vi "art联动采集V4.8.4(导入色码表).vi"() -> ()   [LabVIEW 2016]
uses:
  <vilib>/Utility/file.llb/Read Delimited Spreadsheet (I64).vi
  <vilib>/Instr/_visa.llb/VISA Configure Serial Port (Instr).vi
  <vilib>/Utility/file.llb/Write Delimited Spreadsheet (DBL).vi
panel:
  in  "色码表导入":path caption="（色码表导入）"
  out "水平进度条":u8(slide) scale=0.0..100.0
  out "x+y 3":dbl=3.0
  in  "分层图查看":bool
  in  "hDevice 2":i32
  in  "逐行扫描":bool
  in  "定位模式":bool
  in  "X终点":dbl
  in  "Y终点":dbl
  in  "高级设置":bool
  in  "Y轴回零速度":dbl=15000.0
  in  "X轴回零速度":dbl=15000.0
  in  "细分设置":dbl=8.0
  in  "等待时间":u32=40
  in  "文件保存":path=path "C:/Users/H301/Desktop/art采集实验数据" caption="保存路径"
  out "已用时（s）":dbl
  out "error out":errorcluster caption="错误输出"
  in  "退出扫描(Esc)":bool
  in  "N_Length":i32=16384
  out "M_Length":i32
  out "hDevice":i32=241832032
  out "pulDDR2Length":u32=256
  out "毫秒计时值":u32=3586537
  out "数组":dbl[][](array[numeric])=[[58819.77200735986, 88200.32943600747]]
  out "强度图":dbl[][](graph)=[[58819.77200735986, 88200.32943600747]]
  out "judge":dbl
  out "Xloop":dbl
  out "幅频谱":dbl[](graph)
  out "时域谱":dbl[](graph)
  out "错误输出":errorcluster
  in  "启动":bool
  in  "逐点扫描":bool
  in  "X归零":bool
  in  "Y归零":bool
  in  "Y起点":dbl
  in  "Y轴速度":dbl=9000.0
  in  "X轴速度":dbl=9000.0
  out "电机状态":bool
  in  "电机端口":refnum<visa-resource-name>="COM6"
  out "Yloop":dbl=1.0
  out "X扫描范围":dbl=150.0
  out "Y扫描范围":dbl=75.0
  out "Y序":i32
  in  "X起点":dbl
  out "Y(mm)":dbl
  out "x+y 2":dbl=3.0
  in  "Y:":dbl=1.0
  in  "精度":dbl=0.001
  in  "电机急停":bool
  out "X（mm）":dbl
  out "x+y":dbl=1.0
  in  "X:":dbl=1.0
  # "实时坐标"
  # "时域谱"
  # "频域谱"
  # "归零"
  # "扫描区域"
  # "扫描步进(mm)"
  # "X:"
  # "~"
  # "Y:"
  # "~"
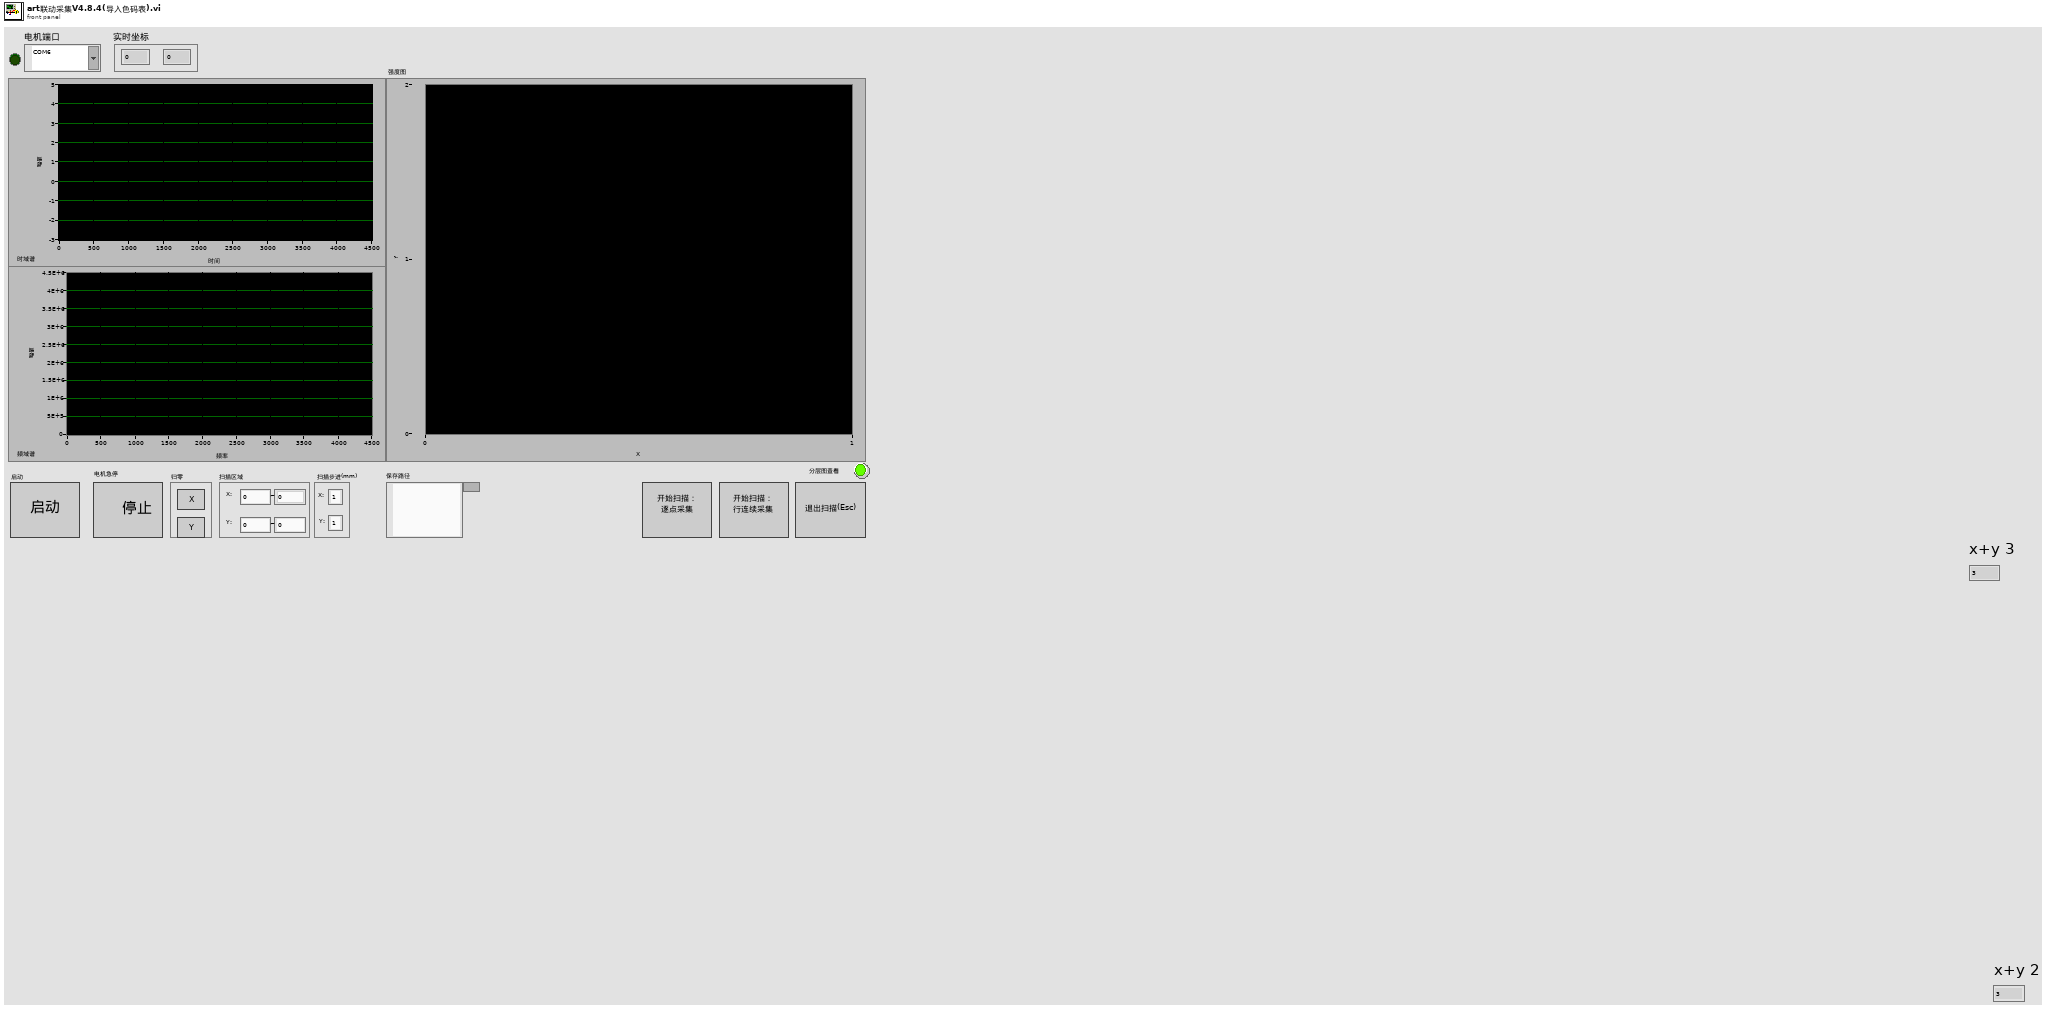
[diagram p1: front panel]
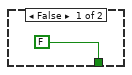
[diagram p2: hidden frame]
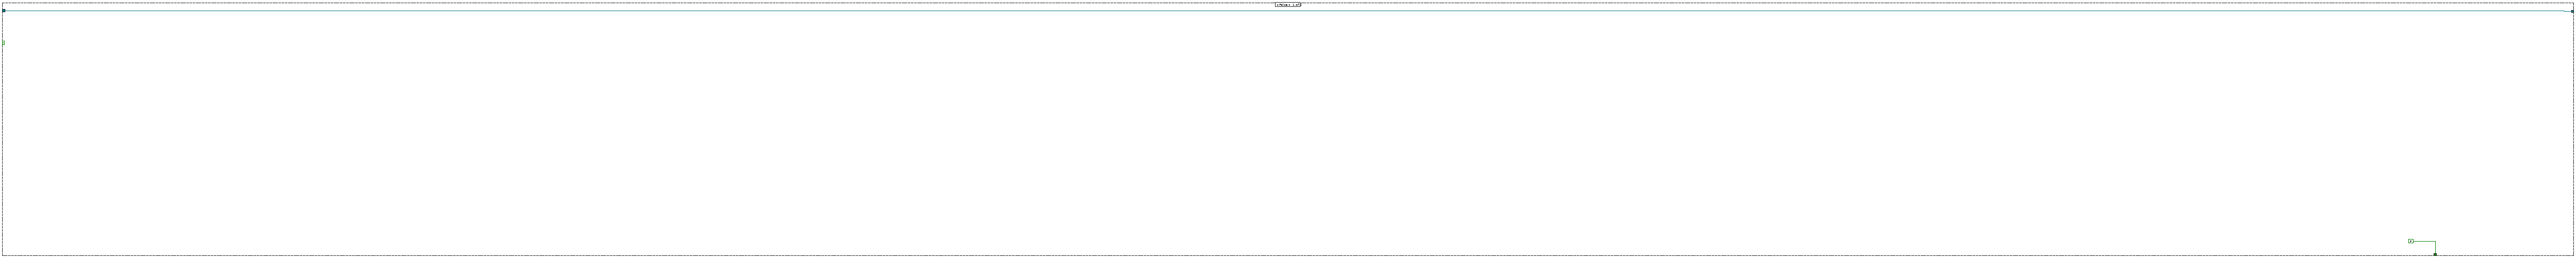
[diagram p3: hidden frame]
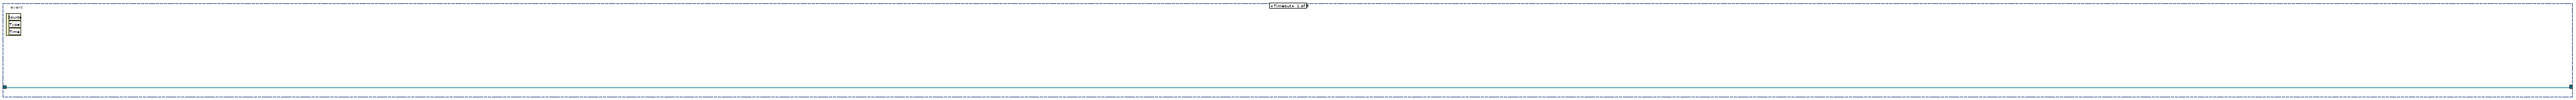
[diagram p4: hidden frame]
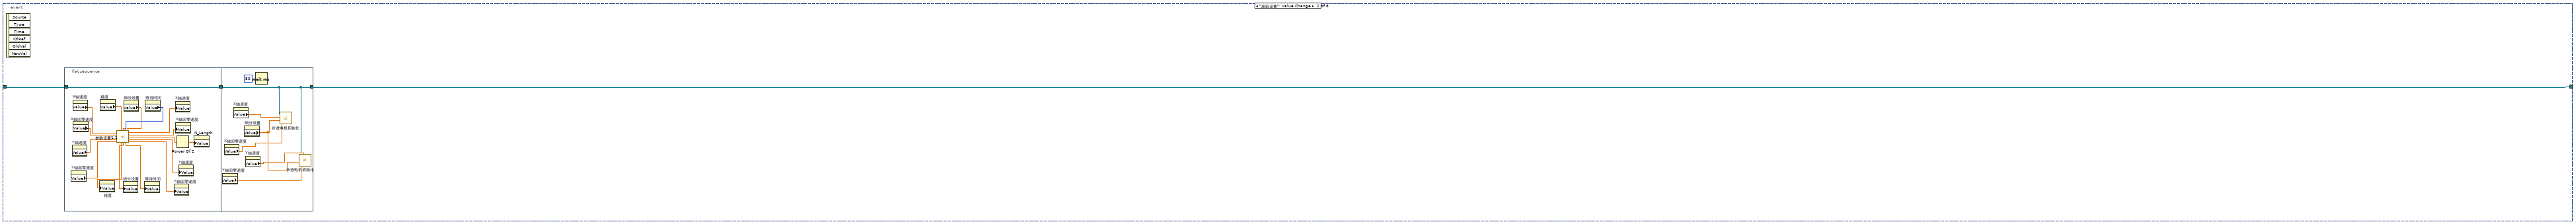
[diagram p5: hidden frame]
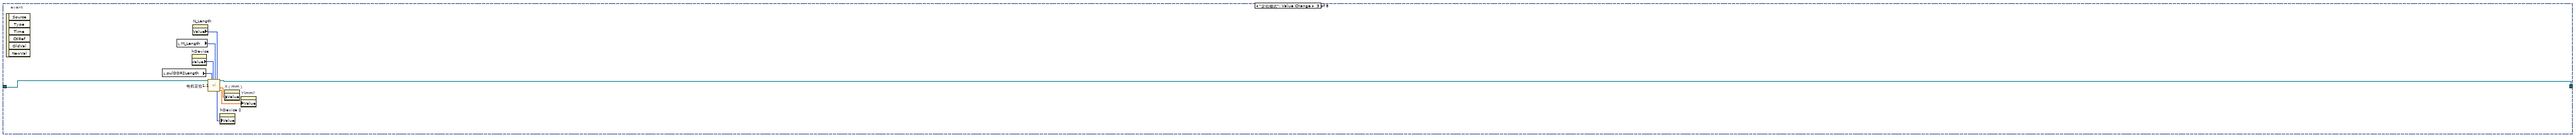
[diagram p6: hidden frame]
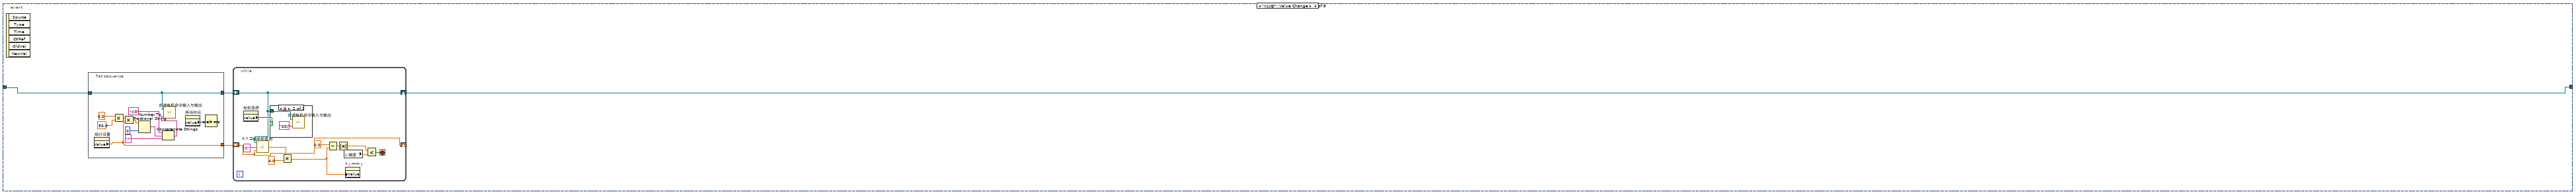
[diagram p7: hidden frame]
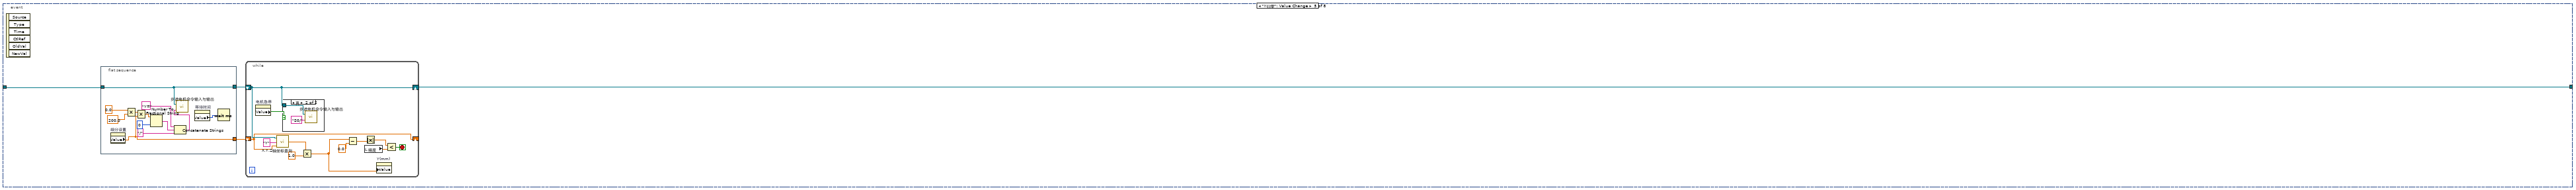
[diagram p9: hidden frame]
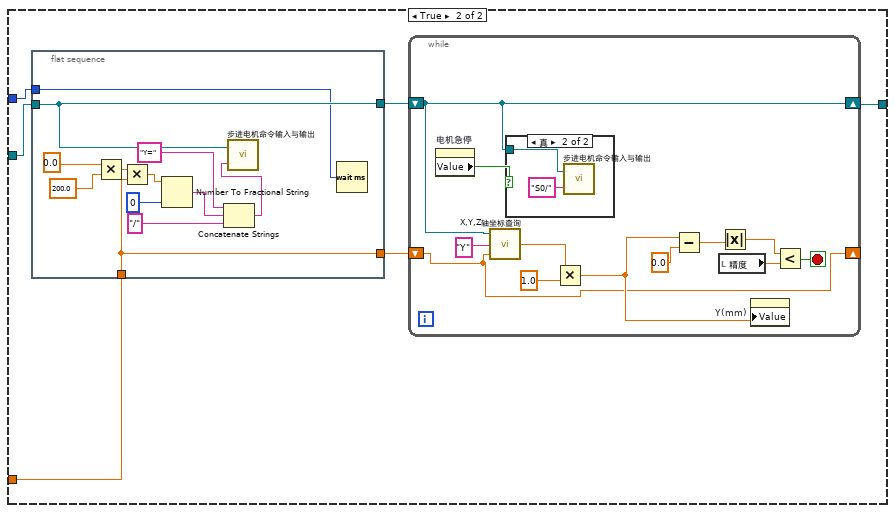
[diagram p15: hidden frame]
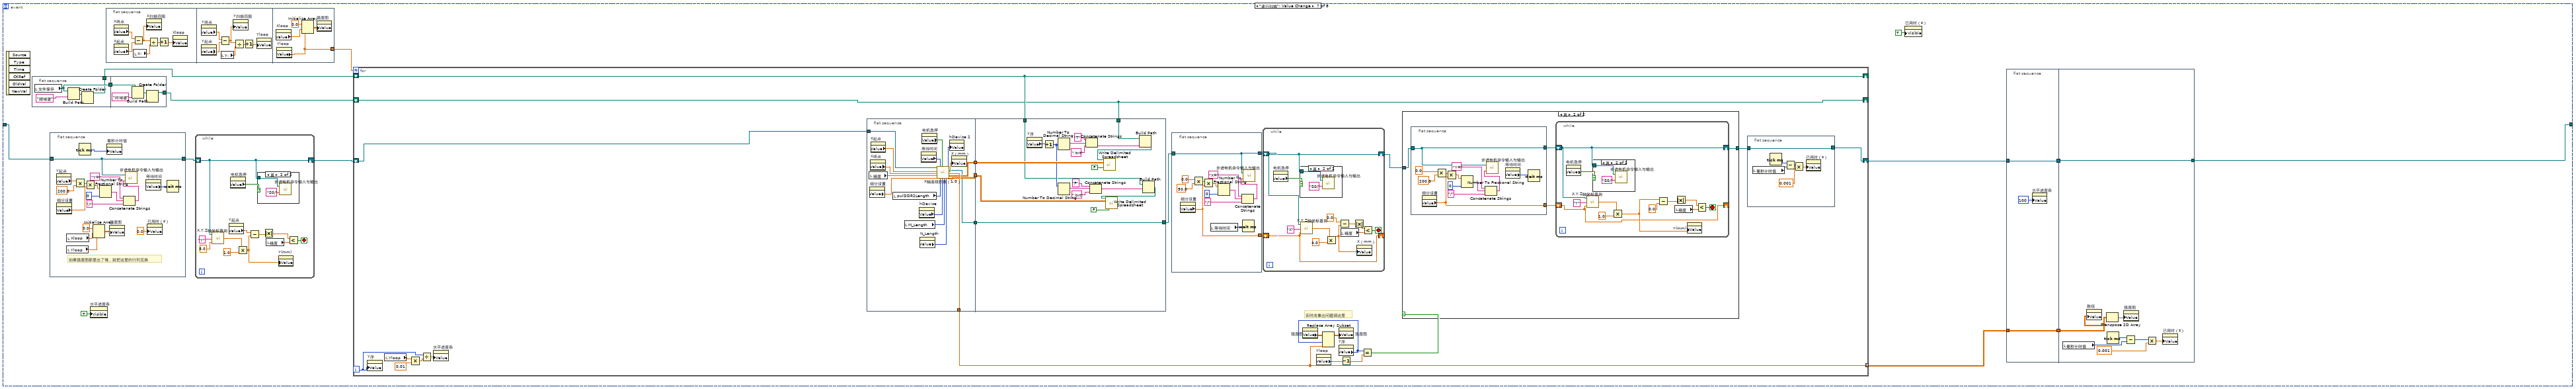
[diagram p19: hidden frame]
diagram:
  n1 = call-poly <vilib>:"Read Delimited Spreadsheet.vi"("file path (dialog if empty)"="色码表导入") -> ("first row"=w1:i64[])  [unwired: 9 in, 5 out]
  n2 = property on="强度图" class="IntGraph (严格)"("Color Table"=w1) -> ()  [unwired: 2 in, 2 out]
  n3 = property on="水平进度条" class="Slide (严格)"("Visible"=FALSE ("可见")) -> ()  [unwired: 2 in, 2 out]
  n4 = while {
    stop <- w7 stop-if-true
    n5 = case shown="真" "启动" {
      tunnel: [FALSE ("ESC") w16] -> w7
      frame False {
      }
      frame True {
        w29 = 0  # OutClockSource
        w30 = 0  # bClockSourceDir
        w32 = 10000000  # Frequency
        w33 = 0  # ClockSource
        w34 = 0  # TrigLevelVolt
        w22 = 1
        w35 = 0  # TriggerDir
        w36 = 0  # TriggerSource
        w37 = 0  # ATRTriggerChannel
        w38 = 0  # TriggerMode
        w23 = 0  # M_Length
        w39 = 1  # CouplingType
        w40 = 0  # DeviceLgcID
        w50 = u16 0 items=["无", "XON/XOFF", "RTS/CTS", "XON/XOFF & RTS/CTS", "DTR/DSR", "XON/XOFF & DTR/DSR"] ("flow control (0:none)")
        w51 = u16 10 items=["1.0"=10, "1.5"=15, "2.0"=20] ("stop bits (10: 1 bit)")
        # "3"
        # "2"
        # "1"
        n6 = call-poly "VISA Configure Serial Port"("VISA resource name"="电机端口", "baud rate (9600)"=u32 9600, "data bits (8)"=u16 8, "parity (0:none)"=enum16{"None", "Odd", "Even", "Mark", "Space"}."None", "stop bits (10: 1 bit)"=w51, "flow control (0:none)"=w50) -> ("VISA resource name out"=w42:refnum<visa-resource-name>, "error out"=→"error out":errorcluster)  [unwired: 1 in, 7 out]
        n7 = Build Array "InputRange"(w22, w22, w22, w22) -> (w21:i32[])
        n8 = dll-call lib="PTH2aabs CUsersH301Desktopart闭环扫描程序采集卡控制INFamd64PCI8502_32.dll" fn="PCI8502_CreateDevice" label="CreateDevice"("DeviceLgcID"=w40) -> (w27:i32)  [unwired: 4 in, 2 out]
        n9 = property on="细分设置" class="DigNum (严格)"() -> ("Value"=w15:dbl)  [unwired: 2 in, 2 out]
        n10 = Build Array (concatenate) "InitDeviceAD"(w32, w21, w39, w23, "N_Length", w38, w37, w36, w35, w34, w33, w30, w29) -> (w31:i32[])
        n11 = call "步进电机初始化.vi"("回零速度"="X轴回零速度", "细分设置"=w15, "X轴速度"="X轴速度", "串口通信端口"=w42) -> ()  [unwired: 2 in, 1 out]
        n12 = dll-call lib="PTH2aabs CUsersH301Desktopart闭环扫描程序采集卡控制INFamd64PCI8502_32.dll" fn="PCI8502_GetDDR2Length" label="GetDDR2Length"("hDevice"=w27, "pulDDR2Length"=u32 0) -> ("hDevice"=w26:i32, "pulDDR2Length"=→"pulDDR2Length":u32)  [unwired: 4 in, 2 out]
        n13 = call "步进电机初始化.vi"("Y轴速度"="Y轴速度", "回零速度"="Y轴回零速度", "细分设置"=w15, "串口通信端口"=w42) -> ()  [unwired: 2 in, 1 out]
        n14 = call "步进电机命令输入与输出.vi"("输入字符串"="?R/", "串口通信端口"=w42) -> ("返回字符串"=w47:string)
        n15 = dll-call lib="PTH2aabs CUsersH301Desktopart闭环扫描程序采集卡控制INFamd64PCI8502_32.dll" fn="PCI8502_InitDeviceAD" label="InitDeviceAD"("hDevice"=w26, "pADPara"=w31) -> ("hDevice"=→"hDevice":i32)  [unwired: 5 in, 2 out]
        n16 = String Subset(string=w47, offset (0)=0 ("偏移量(0)"), length (rest)=2 ("长度（剩余）")) -> (substring=w44:string)
        n17 = Equal?(x=w44, y="OK") -> (x = y?=w41:bool)
        "电机状态" <- w41
        n18 = case shown="真" w41 {
          tunnel: w42 -> [w57 w60]
          tunnel: [w57 w58] -> w17
          tunnel: [FALSE ("ESC") w59] -> w16
          frame False {
          }
          frame True {
            n19 = while {
              tunnel: ["退出扫描(Esc)"] -> w59
              shift-right: [w63] -> w58
              shift-left: w60 -> [w68]
              stop <- "退出扫描(Esc)" stop-if-true
              n20 = property on="水平进度条" class="Slide (严格)"("Visible"=FALSE ("可见")) -> ()  [unwired: 2 in, 2 out]
              n21 = property on="高级设置" class="Bool"("Visible"=TRUE ("可见")) -> ()  [unwired: 2 in, 2 out]
              n22 = property on="定位模式" class="Bool"("Visible"=TRUE ("可见")) -> ()  [unwired: 2 in, 2 out]
              n23 = property on="水平进度条" class="Slide (严格)"("Value"=u8 0 ("水平进度条")) -> ()  [unwired: 2 in, 2 out]
              n24 = event shown="[5] \"逐点扫描\": 值改变" {
                selector: _ -> [_ _ _ _ _ _ _ _]
                dyn-events: _ -> [_ _ _ _ _ _ _ _]
                timeout: 1 -> [_ _ _ _ _ _ _ _]
                tunnel: w68 -> [w69 w72 w105 w109 w139 w190 w499 w727]
                tunnel: [w69 w71 w104 w107 w137 w185 w502 w726] -> w63
                event Timeout {
                  n25 = event-data() -> ()  [unwired: 1 in, 3 out]
                }
                event "高级设置": Value Change {
                  n26 = event-data() -> ()  [unwired: 1 in, 6 out]
                  n27 = flat-sequence {
                    tunnel: w72 -> [w75]
                    tunnel: [w75] -> w70
                    tunnel: [w91] -> w71
                    tunnel: w70 -> [w91]
                    frame #0 {
                      n28 = property on="Y轴回零速度" class="DigNum (严格)"() -> ("Value"=w79:dbl)  [unwired: 2 in, 2 out]
                      n29 = property on="Y轴速度" class="DigNum (严格)"() -> ("Value"=w78:dbl)  [unwired: 2 in, 2 out]
                      n30 = property on="X轴速度" class="DigNum (严格)"() -> ("Value"=w76:dbl)  [unwired: 2 in, 2 out]
                      n31 = property on="X轴回零速度" class="DigNum (严格)"() -> ("Value"=w77:dbl)  [unwired: 2 in, 2 out]
                      n32 = property on="精度" class="DigNum (严格)"() -> ("Value"=w83:dbl)  [unwired: 2 in, 2 out]
                      n33 = property on="细分设置" class="DigNum (严格)"() -> ("Value"=w84:dbl)  [unwired: 2 in, 2 out]
                      n34 = property on="等待时间" class="DigNum (严格)"() -> ("Value"=w85:u32)  [unwired: 2 in, 2 out]
                      n35 = call "参数设置1.1.vi"("X轴速度"=w76, "精度"=w83, "细分设置"=w84, "等待时间"=w85, "X轴回零速度"=w77, "Y轴速度"=w78, "Y轴回零速度"=w79) -> ("X轴速度"=w86:dbl, "X轴回零速度"=w87:dbl, "采样阶"=w73:dbl, "Y轴速度"=w88:dbl, "精度"=w80:dbl, "细分设置"=w81:dbl, "等待时间"=w82:dbl, "Y轴回零速度"=w89:dbl)  [unwired: 1 in]
                      n36 = property on="精度" class="DigNum (严格)"("Value"=w80) -> ()  [unwired: 2 in, 2 out]
                      n37 = property on="细分设置" class="DigNum (严格)"("Value"=w81) -> ()  [unwired: 2 in, 2 out]
                      n38 = property on="等待时间" class="DigNum (严格)"("Value"=w82) -> ()  [unwired: 2 in, 2 out]
                      n39 = property on="Y轴回零速度" class="DigNum (严格)"("Value"=w89) -> ()  [unwired: 2 in, 2 out]
                      n40 = property on="X轴速度" class="DigNum (严格)"("Value"=w86) -> ()  [unwired: 2 in, 2 out]
                      n41 = property on="X轴回零速度" class="DigNum (严格)"("Value"=w87) -> ()  [unwired: 2 in, 2 out]
                      n42 = Power Of 2(x=w73) -> (2^x=w74:dbl)
                      n43 = property on="Y轴速度" class="DigNum (严格)"("Value"=w88) -> ()  [unwired: 2 in, 2 out]
                      n44 = property on="N_Length" class="DigNum (严格)"("Value"=w74) -> ()  [unwired: 2 in, 2 out]
                    }
                    frame #1 {
                      n45 = property on="Y轴回零速度" class="DigNum (严格)"() -> ("Value"=w95:dbl)  [unwired: 2 in, 2 out]
                      n46 = property on="X轴回零速度" class="DigNum (严格)"() -> ("Value"=w94:dbl)  [unwired: 2 in, 2 out]
                      n47 = property on="X轴速度" class="DigNum (严格)"() -> ("Value"=w93:dbl)  [unwired: 2 in, 2 out]
                      n48 = property on="细分设置" class="DigNum (严格)"() -> ("Value"=w92:dbl)  [unwired: 2 in, 2 out]
                      n49 = property on="Y轴速度" class="DigNum (严格)"() -> ("Value"=w96:dbl)  [unwired: 2 in, 2 out]
                      n50 = Wait (ms)(milliseconds to wait=u32 50 ("等待时间（毫秒）")) -> ()  [unwired: 1 out]
                      n51 = call "步进电机初始化.vi"("回零速度"=w94, "细分设置"=w92, "X轴速度"=w93, "串口通信端口"=w91) -> ()  [unwired: 2 in, 1 out]
                      n52 = call "步进电机初始化.vi"("Y轴速度"=w96, "回零速度"=w95, "细分设置"=w92, "串口通信端口"=w91) -> ()  [unwired: 2 in, 1 out]
                    }
                  }
                }
                event "定位模式": Value Change {
                  n53 = event-data() -> ()  [unwired: 1 in, 6 out]
                  n54 = local read "pulDDR2Length"() -> (w101:u32)
                  n55 = local read "M_Length"() -> (w99:i32)
                  n56 = property on="hDevice" class="DigNum (严格)"() -> ("Value"=w100:i32)  [unwired: 2 in, 2 out]
                  n57 = property on="N_Length" class="DigNum (严格)"() -> ("Value"=w98:i32)  [unwired: 2 in, 2 out]
                  n58 = call "电机定位1.1.vi"("VISA I"=w105, "pulDDR2Length"=w101, "hDevice"=w100, "M-length"=w99, "N-length"=w98) -> ("hDevice out"=w97:i32, "VISA O"=w104:refnum<visa-resource-name>, "X"=w103:dbl, "Y"=w102:dbl)  [unwired: 11 in]
                  n59 = property on="hDevice 2" class="DigNum (严格)"("Value"=w97) -> ()  [unwired: 2 in, 2 out]
                  n60 = property on="X（mm）" class="DigNum (严格)"("Value"=w103) -> ()  [unwired: 2 in, 2 out]
                  n61 = property on="Y(mm)" class="DigNum (严格)"("Value"=w102) -> ()  [unwired: 2 in, 2 out]
                }
                event "X归零": Value Change {
                  n62 = event-data() -> ()  [unwired: 1 in, 6 out]
                  n63 = flat-sequence {
                    tunnel: w109 -> [w113]
                    tunnel: [w113] -> w108
                    tunnel: [w110] -> w106
                    frame #0 {
                      n64 = property on="细分设置" class="DigNum (严格)"() -> ("Value"=w110:dbl)  [unwired: 2 in, 2 out]
                      n65 = Multiply(x=0.0, y=50.0) -> (x*y=w116:dbl)
                      n66 = Multiply(x=w116, y=w110) -> (x*y=w121:dbl)
                      n67 = Number To Fractional String(number=w121, precision (6)=i16 0 ("精度(6)")) -> (F-format string=w119:string)  [unwired: 2 out]
                      n68 = Concatenate Strings("X=" ("字符串"), w119, "/" ("字符串")) -> (w114:string)
                      n69 = call "步进电机命令输入与输出.vi"("输入字符串"=w114, "串口通信端口"=w113) -> ()  [unwired: 1 out]
                      n70 = property on="等待时间" class="DigNum (严格)"() -> ("Value"=w111:u32)  [unwired: 2 in, 2 out]
                      n71 = Wait (ms)(milliseconds to wait=w111) -> ()  [unwired: 1 out]
                    }
                  }
                  n72 = while {
                    shift-right: [w123] -> w107
                    shift-left: w108 -> [w123]
                    shift-right: [w122] -> _
                    shift-left: w106 -> [w122]
                    stop <- w129 stop-if-true
                    n73 = property on="电机急停" class="Bool (严格)"() -> ("Value"=w130:bool)  [unwired: 2 in, 2 out]
                    n74 = call "X,Y,Z轴坐标查询.vi"("细分设置"=w122, "查询坐标轴"="X", "串口通信端口"=w123) -> ("坐标(mm)"=w131:dbl)
                    n75 = case shown="真" w130 {
                      tunnel: w123 -> [_ w134]
                      frame False {
                      }
                      frame True {
                        n76 = call "步进电机命令输入与输出.vi"("输入字符串"="S0/", "串口通信端口"=w134) -> ()  [unwired: 1 out]
                      }
                    }
                    n77 = Multiply(x=w131, y=4.0 ("x")) -> (x*y=w127:dbl)
                    n78 = Subtract(x=0.0, y=w127) -> (x-y=w126:dbl)
                    n79 = Absolute Value(x=w126) -> (abs(x)=w125:dbl)
                    n80 = local read "精度"() -> (w128:dbl)
                    n81 = property on="X（mm）" class="DigNum (严格)"("Value"=w127) -> ()  [unwired: 2 in, 2 out]
                    n82 = Less?(x=w125, y=w128) -> (x < y?=w129:bool)
                  }
                }
                event "Y归零": Value Change {
                  n83 = event-data() -> ()  [unwired: 1 in, 6 out]
                  n84 = flat-sequence {
                    tunnel: w139 -> [w143]
                    tunnel: [w143] -> w138
                    tunnel: [w140] -> w136
                    frame #0 {
                      n85 = property on="细分设置" class="DigNum (严格)"() -> ("Value"=w140:dbl)  [unwired: 2 in, 2 out]
                      n86 = Multiply(x=0.0, y=200.0) -> (x*y=w146:dbl)
                      n87 = Multiply(x=w146, y=w140) -> (x*y=w151:dbl)
                      n88 = Number To Fractional String(number=w151, precision (6)=i16 0 ("精度(6)")) -> (F-format string=w149:string)  [unwired: 2 out]
                      n89 = Concatenate Strings("Y=" ("字符串"), w149, "/" ("字符串")) -> (w144:string)
                      n90 = call "步进电机命令输入与输出.vi"("输入字符串"=w144, "串口通信端口"=w143) -> ()  [unwired: 1 out]
                      n91 = property on="等待时间" class="DigNum (严格)"() -> ("Value"=w141:u32)  [unwired: 2 in, 2 out]
                      n92 = Wait (ms)(milliseconds to wait=w141) -> ()  [unwired: 1 out]
                    }
                  }
                  n93 = while {
                    shift-right: [w153] -> w137
                    shift-left: w138 -> [w153]
                    shift-right: [w152] -> _
                    shift-left: w136 -> [w152]
                    stop <- w159 stop-if-true
                    n94 = property on="电机急停" class="Bool (严格)"() -> ("Value"=w160:bool)  [unwired: 2 in, 2 out]
                    n95 = call "X,Y,Z轴坐标查询.vi"("细分设置"=w152, "查询坐标轴"="Y", "串口通信端口"=w153) -> ("坐标(mm)"=w161:dbl)
                    n96 = case shown="真" w160 {
                      tunnel: w153 -> [_ w164]
                      frame False {
                      }
                      frame True {
                        n97 = call "步进电机命令输入与输出.vi"("输入字符串"="S0/", "串口通信端口"=w164) -> ()  [unwired: 1 out]
                      }
                    }
                    n98 = Multiply(x=w161, y=1.0 ("x")) -> (x*y=w157:dbl)
                    n99 = Subtract(x=w157, y=0.0 ("x")) -> (x-y=w155:dbl)
                    n100 = local read "精度"() -> (w158:dbl)
                    n101 = Absolute Value(x=w155) -> (abs(x)=w154:dbl)
                    n102 = property on="Y(mm)" class="DigNum (严格)"("Value"=w157) -> ()  [unwired: 2 in, 2 out]
                    n103 = Less?(x=w154, y=w158) -> (x < y?=w159:bool)
                  }
                }
                event "逐点扫描": Value Change {
                  n104 = event-data() -> ()  [unwired: 1 in, 6 out]
                  n105 = flat-sequence {
                    tunnel: w190 -> [w219]
                    tunnel: [w219] -> w181
                    frame #0 {
                      # "如果强度图那里出了错，就把这里的行列互换"
                      n106 = Tick Count (ms)() -> (millisecond timer value=→"毫秒计时值":u32)
                      n107 = local read "Xloop"() -> (w214:dbl)
                      n108 = local read "Yloop"() -> (w213:dbl)
                      n109 = Multiply(x="Y起点", y=200.0) -> (x*y=w222:dbl)
                      n110 = Multiply(x=w222, y="细分设置") -> (x*y=w227:dbl)
                      n111 = Initialize Array(0.0 ("元素"), w214, w213) -> (→"强度图":dbl[][])
                      n112 = Number To Fractional String(number=w227, precision (6)=i16 0 ("精度(6)")) -> (F-format string=w225:string)  [unwired: 2 out]
                      n113 = Concatenate Strings("Y=" ("字符串"), w225, "/" ("字符串")) -> (w220:string)
                      n114 = call "步进电机命令输入与输出.vi"("输入字符串"=w220, "串口通信端口"=w219) -> ()  [unwired: 1 out]
                      n115 = property on="已用时（s）" class="DigNum (严格)"("Value"=0.0 ("已用时（s）")) -> ()  [unwired: 2 in, 2 out]
                      n116 = property on="等待时间" class="DigNum (严格)"() -> ("Value"=w211:u32)  [unwired: 2 in, 2 out]
                      n117 = Wait (ms)(milliseconds to wait=w211) -> ()  [unwired: 1 out]
                    }
                  }
                  n118 = local read "X起点"() -> (w177:dbl)
                  n119 = property on="水平进度条" class="Slide (严格)"("Visible"=TRUE ("可见")) -> ()  [unwired: 2 in, 2 out]
                  n120 = Subtract(x="X终点", y=w177) -> (x-y=w176:dbl)
                  "X扫描范围" <- w176
                  n121 = local read "X:"() -> (w184:dbl)
                  n122 = Divide(x=w176, y=w184) -> (x/y=w182:dbl)
                  n123 = Increment(x=w182) -> (x+1=→"Xloop":dbl)
                  n124 = while {
                    shift-right: [w228] -> w173
                    shift-left: w181 -> [w228]
                    stop <- w233 stop-if-true
                    n125 = call "X,Y,Z轴坐标查询.vi"("细分设置"=8.0, "查询坐标轴"="Y", "串口通信端口"=w228) -> ("坐标(mm)"=w235:dbl)
                    n126 = property on="Y起点" class="DigNum (严格)"() -> ("Value"=w237:dbl)  [unwired: 2 in, 2 out]
                    n127 = property on="电机急停" class="Bool (严格)"() -> ("Value"=w234:bool)  [unwired: 2 in, 2 out]
                    n128 = Multiply(x=w235, y=1.0 ("x")) -> (x*y=w231:dbl)
                    n129 = Subtract(x=w237, y=w231) -> (x-y=w230:dbl)
                    n130 = case shown="真" w234 {
                      tunnel: w228 -> [_ w240]
                      frame False {
                      }
                      frame True {
                        n131 = call "步进电机命令输入与输出.vi"("输入字符串"="S0/", "串口通信端口"=w240) -> ()  [unwired: 1 out]
                      }
                    }
                    n132 = Absolute Value(x=w230) -> (abs(x)=w229:dbl)
                    n133 = local read "精度"() -> (w232:dbl)
                    n134 = property on="Y(mm)" class="DigNum (严格)"("Value"=w231) -> ()  [unwired: 2 in, 2 out]
                    n135 = Less?(x=w229, y=w232) -> (x < y?=w233:bool)
                  }
                  n136 = local read "Y起点"() -> (w179:dbl)
                  n137 = Subtract(x="Y终点", y=w179) -> (x-y=w175:dbl)
                  "Y扫描范围" <- w175
                  n138 = local read "Y:"() -> (w189:dbl)
                  n139 = Divide(x=w175, y=w189) -> (x/y=w188:dbl)
                  n140 = Increment(x=w188) -> (x+1=w187:dbl)
                  "Yloop" <- w187
                  n141 = for {
                    N: w187 -> [_]
                    shift-right: [w265] -> w166
                    shift-left: w173 -> [w246]
                    tunnel: [w248] -> w186 mode=indexing
                    tunnel: w171 -> [w252]
                    tunnel: w174 -> [w251]
                    i -> [w266]
                    # "实时成像出问题调这里"
                    n142 = flat-sequence {
                      tunnel: w246 -> [w323]
                      tunnel: [w323] -> w264
                      tunnel: [w322] -> w256
                      frame #0 {
                        n143 = property on="X起点" class="DigNum (严格)"() -> ("Value"=w320:dbl)  [unwired: 2 in, 2 out]
                        n144 = property on="细分设置" class="DigNum (严格)"() -> ("Value"=w322:dbl)  [unwired: 2 in, 2 out]
                        n145 = local read "等待时间"() -> (w321:u32)
                        n146 = Multiply(x=w320, y=50.0) -> (x*y=w326:dbl)
                        n147 = Multiply(x=w326, y=w322) -> (x*y=w331:dbl)
                        n148 = Wait (ms)(milliseconds to wait=w321) -> ()  [unwired: 1 out]
                        n149 = Number To Fractional String(number=w331, precision (6)=i16 0 ("精度(6)")) -> (F-format string=w329:string)  [unwired: 2 out]
                        n150 = Concatenate Strings("X=" ("字符串"), w329, "/" ("字符串")) -> (w324:string)
                        n151 = call "步进电机命令输入与输出.vi"("输入字符串"=w324, "串口通信端口"=w323) -> ()  [unwired: 1 out]
                      }
                    }
                    n152 = while {
                      shift-right: [w333] -> w244
                      shift-left: w264 -> [w333]
                      shift-right: [w332] -> _
                      shift-left: w256 -> [w332]
                      stop <- w338 stop-if-true
                      n153 = property on="电机急停" class="Bool (严格)"() -> ("Value"=w339:bool)  [unwired: 2 in, 2 out]
                      n154 = case shown="真" w339 {
                        tunnel: w333 -> [_ w344]
                        frame False {
                        }
                        frame True {
                          n155 = call "步进电机命令输入与输出.vi"("输入字符串"="S0/", "串口通信端口"=w344) -> ()  [unwired: 1 out]
                        }
                      }
                      n156 = call "X,Y,Z轴坐标查询.vi"("细分设置"=w332, "查询坐标轴"="X", "串口通信端口"=w333) -> ("坐标(mm)"=w340:dbl)
                      n157 = Multiply(x=w340, y=4.0 ("x")) -> (x*y=w336:dbl)
                      n158 = property on="X起点" class="DigNum (严格)"() -> ("Value"=w342:dbl)  [unwired: 2 in, 2 out]
                      n159 = Subtract(x=w342, y=w336) -> (x-y=w335:dbl)
                      n160 = Absolute Value(x=w335) -> (abs(x)=w334:dbl)
                      n161 = local read "精度"() -> (w337:dbl)
                      n162 = property on="X（mm）" class="DigNum (严格)"("Value"=w336) -> ()  [unwired: 2 in, 2 out]
                      n163 = Less?(x=w334, y=w337) -> (x < y?=w338:bool)
                    }
                    n164 = local read "Xloop"() -> (w257:dbl)
                    n165 = for {
                      N: w257 -> [_]
                      shift-right: [w427] -> w245
                      shift-left: w244 -> [w423]
                      tunnel: [w426] -> w263 mode=indexing
                      tunnel: [w425] -> w262 mode=indexing
                      tunnel: [w424] -> w248 mode=indexing
                      i -> [w415]
                      n166 = flat-sequence {
                        tunnel: w423 -> [w432]
                        tunnel: [w431] -> w428
                        tunnel: w415 -> [w429]
                        tunnel: [w490] -> w427
                        tunnel: w428 -> [w490]
                        tunnel: [w489] -> w426
                        tunnel: [w488] -> w425
                        tunnel: [w486] -> w424
                        frame #0 {
                          n167 = Equal To 0?(x=w429) -> (x = 0?=w430:bool)
                          n168 = case shown="假" w430 {
                            tunnel: w432 -> [w435 w470]
                            tunnel: [w434 w470] -> w431
                            frame False {
                              n169 = flat-sequence {
                                tunnel: w435 -> [w445]
                                tunnel: [w445] -> w436
                                tunnel: [w437] -> w433
                                frame #0 {
                                n170 = local read "X:"() -> (w439:dbl)
                                n171 = Multiply(x=w439, y=1.0 ("x")) -> (x*y=w444:dbl)
                                n172 = property on="等待时间" class="DigNum (严格)"() -> ("Value"=w438:u32)  [unwired: 2 in, 2 out]
                                n173 = property on="细分设置" class="DigNum (严格)"() -> ("Value"=w437:dbl)  [unwired: 2 in, 2 out]
                                n174 = call "X,Y,Z轴坐标查询.vi"("细分设置"=w437, "查询坐标轴"="X", "串口通信端口"=w445) -> ("坐标(mm)"=w441:dbl)
                                n175 = Multiply(x=4.0, y=w441) -> (x*y=w440:dbl)
                                n176 = Add(x=w440, y=w444) -> (x+y=w447:dbl)
                                "x+y" <- w447
                                n177 = Multiply(x=w447, y=50.0) -> (x*y=w450:dbl)
                                n178 = Multiply(x=w450, y=w437) -> (x*y=w455:dbl)
                                n179 = Number To Fractional String(number=w455, precision (6)=i16 0 ("精度(6)")) -> (F-format string=w453:string)  [unwired: 2 out]
                                n180 = Concatenate Strings("X=" ("字符串"), w453, "/" ("字符串")) -> (w448:string)
                                n181 = call "步进电机命令输入与输出.vi"("输入字符串"=w448, "串口通信端口"=w445) -> ()  [unwired: 1 out]
                                n182 = Wait (ms)(milliseconds to wait=w438) -> ()  [unwired: 1 out]
                                }
                              }
                              n183 = while {
                                shift-right: [w465] -> w434
                                shift-left: w436 -> [w465]
                                shift-right: [w456] -> _
                                shift-left: w433 -> [w456]
                                stop <- w464 stop-if-true
                                n184 = property on="电机急停" class="Bool (严格)"() -> ("Value"=w462:bool)  [unwired: 2 in, 2 out]
                                n185 = local read "x+y"() -> (w466:dbl)
                                n186 = case shown="真" w462 {
                                tunnel: w465 -> [_ w468]
                                frame False {
                                }
                                frame True {
                                n187 = call "步进电机命令输入与输出.vi"("输入字符串"="S0/", "串口通信端口"=w468) -> ()  [unwired: 1 out]
                                }
                                }
                                n188 = call "X,Y,Z轴坐标查询.vi"("细分设置"=w456, "查询坐标轴"="X", "串口通信端口"=w465) -> ("坐标(mm)"=w460:dbl)
                                n189 = Multiply(x=4.0, y=w460) -> (x*y=w459:dbl)
                                n190 = Subtract(x=w466, y=w459) -> (x-y=w458:dbl)
                                n191 = property on="X（mm）" class="DigNum (严格)"("Value"=w459) -> ()  [unwired: 2 in, 2 out]
                                n192 = Absolute Value(x=w458) -> (abs(x)=w457:dbl)
                                n193 = local read "精度"() -> (w461:dbl)
                                n194 = Less?(x=w457, y=w461) -> (x < y?=w464:bool)
                              }
                            }
                            frame True {
                            }
                          }
                        }
                        frame #1 {
                          n195 = local read "pulDDR2Length"() -> (w485:u32)
                          n196 = local read "M_Length"() -> (w484:i32)
                          n197 = property on="N_Length" class="DigNum (严格)"() -> ("Value"=w473:i32)  [unwired: 2 in, 2 out]
                          n198 = Subtract(x=w473, y=w484) -> (x-y=w482:i32)
                          n199 = property on="hDevice" class="DigNum (严格)"() -> ("Value"=w471:i32)  [unwired: 2 in, 2 out]
                          n200 = Multiply(x=w482, y=0.25) -> (x*y=w475:dbl)
                          n201 = Multiply(x=w475, y=0.442) -> (x*y=w477:dbl)
                          n202 = Multiply(x=w475, y=0.058) -> (x*y=w479:dbl)
                          n203 = Round Toward -Infinity(1:w477) -> (0:w474:dbl)
                          n204 = Round Toward -Infinity(1:w479) -> (0:w478:dbl)
                          n205 = call "AD（V3.2）.vi"("N-length"=w473, "M-length"=w484, "hDevice"=w471, "pulDDR2Length"=w485) -> ("幅频谱"=w488:dbl[], "时域谱"=w489:dbl[], "hDevice out"=w472:i32)  [unwired: 5 in]
                          "时域谱" <- w489
                          "幅频谱" <- w488
                          n206 = Increment(x=w474) -> (x+1=w481:dbl)
                          n207 = property on="hDevice 2" class="DigNum (严格)"("Value"=w472) -> ()  [unwired: 2 in, 2 out]
                          n208 = Array Subset(array=w488, index=w478, length=w481) -> (w487:dbl[])
                          n209 = Array Max & Min(array=w487) -> (max value=w486:dbl)  [unwired: 3 out]
                        }
                      }
                      n210 = local read "Y序"() -> (w417:i32)
                      n211 = local read "Xloop"() -> (w418:dbl)
                      n212 = Multiply(x=w417, y=w418) -> (x*y=w416:dbl)
                      n213 = Add(x=w415, y=w416) -> (x+y=w414:dbl)
                      n214 = Multiply(x=w414, y=100.0) -> (x*y=w412:dbl)
                      n215 = local read "Xloop"() -> (w422:dbl)
                      n216 = local read "Yloop"() -> (w421:dbl)
                      n217 = Multiply(x=w421, y=w422) -> (x*y=w420:dbl)
                      n218 = Divide(x=w412, y=w420) -> (x/y=→"水平进度条":dbl)
                    }
                    n219 = flat-sequence {
                      tunnel: w262 -> [w306]
                      tunnel: w263 -> [w314]
                      tunnel: w245 -> [w318]
                      tunnel: [w318] -> w258
                      tunnel: w252 -> [w301]
                      tunnel: w251 -> [w300]
                      frame #0 {
                        n220 = local read "Y序"() -> (w302:i32)
                        n221 = Increment(x=w302) -> (x+1=w303:i32)
                        n222 = Number To Decimal String(number=w303) -> (decimal integer string=w312:string)  [unwired: 1 in]
                        n223 = Number To Decimal String(number=w303) -> (decimal integer string=w311:string)  [unwired: 1 in]
                        n224 = Concatenate Strings("T" ("字符串"), w312, ".txt" ("字符串")) -> (w315:string)
                        n225 = Concatenate Strings("F" ("字符串"), w311, ".txt" ("字符串")) -> (w309:string)
                        n226 = Build Path(base path=w301, name or relative path=w315) -> (appended path=w317:path)
                        n227 = call-poly <vilib>:"Write Delimited Spreadsheet.vi"("file path (dialog if empty)"=w317, "2D data"=w314, "transpose? (no:F)"=FALSE) -> ()  [unwired: 11 in, 2 out]
                        n228 = Build Path(base path=w300, name or relative path=w309) -> (appended path=w307:path)
                        n229 = call-poly <vilib>:"Write Delimited Spreadsheet.vi"("file path (dialog if empty)"=w307, "2D data"=w306, "transpose? (no:F)"=FALSE) -> ()  [unwired: 11 in, 2 out]
                        "judge" <- 1.0
                      }
                    }
                    n230 = flat-sequence {
                      tunnel: w258 -> [w277]
                      tunnel: [w277] -> w259
                      tunnel: [w275] -> w255
                      frame #0 {
                        n231 = property on="细分设置" class="DigNum (严格)"() -> ("Value"=w275:dbl)  [unwired: 2 in, 2 out]
                        n232 = property on="等待时间" class="DigNum (严格)"() -> ("Value"=w274:u32)  [unwired: 2 in, 2 out]
                        n233 = Multiply(x=0.0, y=50.0) -> (x*y=w280:dbl)
                        n234 = Multiply(x=w280, y=w275) -> (x*y=w285:dbl)
                        n235 = Wait (ms)(milliseconds to wait=w274) -> ()  [unwired: 1 out]
                        n236 = Number To Fractional String(number=w285, precision (6)=i16 0 ("精度(6)")) -> (F-format string=w283:string)  [unwired: 2 out]
                        n237 = Concatenate Strings("X=" ("字符串"), w283, "/" ("字符串")) -> (w278:string)
                        n238 = call "步进电机命令输入与输出.vi"("输入字符串"=w278, "串口通信端口"=w277) -> ()  [unwired: 1 out]
                      }
                    }
                    n239 = while {
                      shift-right: [w287] -> w243
                      shift-left: w259 -> [w287]
                      shift-right: [w286] -> _
                      shift-left: w255 -> [w286]
                      stop <- w293 stop-if-true
                      n240 = property on="电机急停" class="Bool (严格)"() -> ("Value"=w294:bool)  [unwired: 2 in, 2 out]
                      n241 = call "X,Y,Z轴坐标查询.vi"("细分设置"=w286, "查询坐标轴"="X", "串口通信端口"=w287) -> ("坐标(mm)"=w295:dbl)
                      n242 = case shown="真" w294 {
                        tunnel: w287 -> [_ w298]
                        frame False {
                        }
                        frame True {
                          n243 = call "步进电机命令输入与输出.vi"("输入字符串"="S0/", "串口通信端口"=w298) -> ()  [unwired: 1 out]
                        }
                      }
                      n244 = Multiply(x=w295, y=4.0 ("x")) -> (x*y=w291:dbl)
                      n245 = Subtract(x=0.0, y=w291) -> (x-y=w290:dbl)
                      n246 = Absolute Value(x=w290) -> (abs(x)=w289:dbl)
                      n247 = local read "精度"() -> (w292:dbl)
                      n248 = property on="X（mm）" class="DigNum (严格)"("Value"=w291) -> ()  [unwired: 2 in, 2 out]
                      n249 = Less?(x=w289, y=w292) -> (x < y?=w293:bool)
                    }
                    n250 = property on="强度图" class="IntGraph (严格)"() -> ("Value"=w249:dbl[][])  [unwired: 2 in, 2 out]
                    n251 = local read "Yloop"() -> (w260:dbl)
                    n252 = Decrement(x=w260) -> (x-1=w261:dbl)
                    n253 = local read "Y序"() -> (w247:i32)
                    n254 = Replace Array Subset(array=w249, new element=w248, index (col)=w247) -> (w250:dbl[][])  [unwired: 1 in]
                    n255 = property on="强度图" class="IntGraph (严格)"("Value"=w250) -> ()  [unwired: 2 in, 2 out]
                    n256 = Equal?(x=w247, y=w261) -> (x = y?=w267:bool)
                    n257 = Increment(x=w247) -> ()  [unwired: 1 out]
                    n258 = flat-sequence {
                      tunnel: w243 -> [w273]
                      tunnel: [w273] -> w242
                      frame #0 {
                        n259 = local read "毫秒计时值"() -> (w268:u32)
                        n260 = Tick Count (ms)() -> (millisecond timer value=w272:u32)
                        n261 = Subtract(x=w272, y=w268) -> (x-y=w269:u32)
                        n262 = Multiply(x=w269, y=0.001) -> (x*y=→"已用时（s）":dbl)
                      }
                    }
                    n263 = property on="细分设置" class="DigNum (严格)"() -> ("Value"=w253:dbl)  [unwired: 2 in, 2 out]
                    n264 = property on="等待时间" class="DigNum (严格)"() -> ("Value"=w254:u32)  [unwired: 2 in, 2 out]
                    n265 = case shown="假" w267 {
                      tunnel: w242 -> [w351 w383]
                      tunnel: [w349 w384] -> w265
                      tunnel: w254 -> [w347 w381]
                      tunnel: w253 -> [w346 w380]
                      frame False {
                        n266 = flat-sequence {
                          tunnel: w351 -> [w355]
                          tunnel: [w355] -> w350
                          tunnel: [w353] -> w348
                          tunnel: w347 -> [w354]
                          tunnel: w346 -> [w353]
                          frame #0 {
                            n267 = call "X,Y,Z轴坐标查询.vi"("细分设置"=w353, "查询坐标轴"="Y", "串口通信端口"=w355) -> ("坐标(mm)"=w356:dbl)
                            n268 = property on="Y:" class="DigNum (严格)"() -> ("Value"=w352:dbl)  [unwired: 2 in, 2 out]
                            n269 = Add(x=w356, y=w352) -> (x+y=w358:dbl)
                            "x+y 2" <- w358
                            n270 = Multiply(x=w358, y=200.0) -> (x*y=w362:dbl)
                            n271 = Multiply(x=w362, y=8.0 ("细分设置")) -> (x*y=w367:dbl)
                            n272 = Number To Fractional String(number=w367, precision (6)=i16 0 ("精度(6)")) -> (F-format string=w365:string)  [unwired: 2 out]
                            n273 = Concatenate Strings("Y=" ("字符串"), w365, "/" ("字符串")) -> (w360:string)
                            n274 = call "步进电机命令输入与输出.vi"("输入字符串"=w360, "串口通信端口"=w355) -> ()  [unwired: 1 out]
                            n275 = Wait (ms)(milliseconds to wait=w354) -> ()  [unwired: 1 out]
                          }
                        }
                        n276 = while {
                          shift-right: [w369] -> w349
                          shift-left: w350 -> [w369]
                          shift-right: [w368] -> _
                          shift-left: w348 -> [w368]
                          stop <- w375 stop-if-true
                          n277 = call "X,Y,Z轴坐标查询.vi"("细分设置"=w368, "查询坐标轴"="Y", "串口通信端口"=w369) -> ("坐标(mm)"=w373:dbl)
                          n278 = local read "x+y 2"() -> (w376:dbl)
                          n279 = property on="电机急停" class="Bool (严格)"() -> ("Value"=w372:bool)  [unwired: 2 in, 2 out]
                          n280 = property on="Y(mm)" class="DigNum (严格)"("Value"=w373) -> ()  [unwired: 2 in, 2 out]
                          n281 = case shown="真" w372 {
                            tunnel: w369 -> [_ w378]
                            frame False {
                            }
                            frame True {
                              n282 = call "步进电机命令输入与输出.vi"("输入字符串"="S0/", "串口通信端口"=w378) -> ()  [unwired: 1 out]
                            }
                          }
                          n283 = Subtract(x=w376, y=w373) -> (x-y=w371:dbl)
                          n284 = Absolute Value(x=w371) -> (abs(x)=w370:dbl)
                          n285 = local read "精度"() -> (w374:dbl)
                          n286 = Less?(x=w370, y=w374) -> (x < y?=w375:bool)
                        }
                      }
                      frame True {
                        n287 = flat-sequence {
                          tunnel: [w388] -> _
                          tunnel: [w388] -> w385
                          tunnel: w383 -> [w388]
                          tunnel: [w386] -> w382
                          tunnel: w381 -> [w387]
                          tunnel: w380 -> [w386]
                          frame #0 {
                            n288 = Multiply(x=0.0, y=200.0) -> (x*y=w392:dbl)
                            n289 = Multiply(x=w392, y=w386) -> (x*y=w397:dbl)
                            n290 = Number To Fractional String(number=w397, precision (6)=i16 0 ("精度(6)")) -> (F-format string=w395:string)  [unwired: 2 out]
                            n291 = Concatenate Strings("Y=" ("字符串"), w395, "/" ("字符串")) -> (w390:string)
                            n292 = call "步进电机命令输入与输出.vi"("输入字符串"=w390, "串口通信端口"=w388) -> ()  [unwired: 1 out]
                            n293 = Wait (ms)(milliseconds to wait=w387) -> ()  [unwired: 1 out]
                          }
                        }
                        n294 = while {
                          shift-right: [w399] -> w384
                          shift-left: w385 -> [w399]
                          shift-right: [w398] -> _
                          shift-left: w382 -> [w398]
                          stop <- w405 stop-if-true
                          n295 = property on="电机急停" class="Bool (严格)"() -> ("Value"=w406:bool)  [unwired: 2 in, 2 out]
                          n296 = call "X,Y,Z轴坐标查询.vi"("细分设置"=w398, "查询坐标轴"="Y", "串口通信端口"=w399) -> ("坐标(mm)"=w407:dbl)
                          n297 = case shown="真" w406 {
                            tunnel: w399 -> [_ w410]
                            frame False {
                            }
                            frame True {
                              n298 = call "步进电机命令输入与输出.vi"("输入字符串"="S0/", "串口通信端口"=w410) -> ()  [unwired: 1 out]
                            }
                          }
                          n299 = Multiply(x=w407, y=1.0 ("x")) -> (x*y=w403:dbl)
                          n300 = Subtract(x=w403, y=0.0 ("x")) -> (x-y=w401:dbl)
                          n301 = local read "精度"() -> (w404:dbl)
                          n302 = Absolute Value(x=w401) -> (abs(x)=w400:dbl)
                          n303 = property on="Y(mm)" class="DigNum (严格)"("Value"=w403) -> ()  [unwired: 2 in, 2 out]
                          n304 = Less?(x=w400, y=w404) -> (x < y?=w405:bool)
                        }
                      }
                    }
                    "Y序" <- w266
                  }
                  n305 = property on="已用时（s）" class="DigNum (严格)"("Visible"=TRUE ("可见")) -> ()  [unwired: 2 in, 2 out]
                  n306 = flat-sequence {
                    tunnel: [w191] -> w174
                    tunnel: ["文件保存"] -> w172
                    tunnel: w172 -> [w196]
                    tunnel: [w195] -> w171
                    frame #0 {
                      n307 = Build Path(base path="文件保存", name or relative path="频域谱" ("名称或相对路径")) -> (appended path=w194:path)
                      n308 = Create Folder(path (use dialog)=w194) -> (created path=w191:path)  [unwired: 2 in, 2 out]
                    }
                    frame #1 {
                      n309 = Build Path(base path=w196, name or relative path="时域谱" ("名称或相对路径")) -> (appended path=w197:path)
                      n310 = Create Folder(path (use dialog)=w197) -> (created path=w195:path)  [unwired: 2 in, 2 out]
                    }
                  }
                  n311 = flat-sequence {
                    tunnel: w186 -> [w201]
                    tunnel: [w199] -> _
                    tunnel: [w199] -> w168
                    tunnel: [w201] -> w167
                    tunnel: w166 -> [w199]
                    tunnel: [w202] -> w185
                    tunnel: w168 -> [w202]
                    tunnel: w167 -> [w205]
                    frame #0 {
                      n312 = property on="水平进度条" class="Slide (严格)"("Value"=u8 100 ("水平进度条")) -> ()  [unwired: 2 in, 2 out]
                    }
                    frame #1 {
                      n313 = local read "毫秒计时值"() -> (w204:u32)
                      n314 = Tick Count (ms)() -> (millisecond timer value=w209:u32)
                      n315 = Transpose 2D Array(2D array=w205) -> (transposed array=w206:dbl[][])
                      n316 = Subtract(x=w209, y=w204) -> (x-y=w207:u32)
                      n317 = property on="强度图" class="IntGraph (严格)"("Value"=w206) -> ()  [unwired: 2 in, 2 out]
                      n318 = Multiply(x=w207, y=0.001) -> (x*y=w203:dbl)
                      n319 = property on="已用时（s）" class="DigNum (严格)"("Value"=w203) -> ()  [unwired: 2 in, 2 out]
                      "数组" <- w205
                    }
                  }
                }
                event "逐行扫描": Value Change {
                  n320 = event-data() -> ()  [unwired: 1 in, 6 out]
                  n321 = flat-sequence {
                    tunnel: [w565] -> w504
                    tunnel: [w564] -> w501
                    tunnel: w504 -> [w569]
                    tunnel: [w568] -> w503
                    frame #0 {
                      n322 = local read "文件保存"() -> (w565:path)
                      n323 = Build Path(base path=w565, name or relative path="频域谱" ("名称或相对路径")) -> (appended path=w567:path)
                      n324 = Create Folder(path (use dialog)=w567) -> (created path=w564:path)  [unwired: 2 in, 2 out]
                    }
                    frame #1 {
                      n325 = Build Path(base path=w569, name or relative path="时域谱" ("名称或相对路径")) -> (appended path=w570:path)
                      n326 = Create Folder(path (use dialog)=w570) -> (created path=w568:path)  [unwired: 2 in, 2 out]
                    }
                  }
                  n327 = flat-sequence {
                    tunnel: w499 -> [w522]
                    tunnel: [w522] -> w498
                    frame #0 {
                      # "如果强度图那里出了错，就把这里的行列互换"
                      n328 = property on="Y起点" class="DigNum (严格)"() -> ("Value"=w525:dbl)  [unwired: 2 in, 2 out]
                      n329 = property on="细分设置" class="DigNum (严格)"() -> ("Value"=w523:dbl)  [unwired: 2 in, 2 out]
                      n330 = local read "Xloop"() -> (w529:dbl)
                      n331 = local read "Yloop"() -> (w528:dbl)
                      n332 = Multiply(x=w525, y=200.0) -> (x*y=w533:dbl)
                      n333 = Tick Count (ms)() -> (millisecond timer value=w526:u32)
                      n334 = Multiply(x=w533, y=w523) -> (x*y=w538:dbl)
                      n335 = Initialize Array(0.0 ("元素"), w529, w528) -> (w524:dbl[][])
                      n336 = Number To Fractional String(number=w538, precision (6)=i16 0 ("精度(6)")) -> (F-format string=w536:string)  [unwired: 2 out]
                      n337 = property on="毫秒计时值" class="DigNum (严格)"("Value"=w526) -> ()  [unwired: 2 in, 2 out]
                      n338 = property on="强度图" class="IntGraph (严格)"("Value"=w524) -> ()  [unwired: 2 in, 2 out]
                      n339 = Concatenate Strings("Y=" ("字符串"), w536, "/" ("字符串")) -> (w531:string)
                      n340 = call "步进电机命令输入与输出.vi"("输入字符串"=w531, "串口通信端口"=w522) -> ()  [unwired: 1 out]
                      n341 = property on="等待时间" class="DigNum (严格)"() -> ("Value"=w527:u32)  [unwired: 2 in, 2 out]
                      n342 = property on="已用时（s）" class="DigNum (严格)"("Value"=0.0 ("已用时（s）")) -> ()  [unwired: 2 in, 2 out]
                      n343 = Wait (ms)(milliseconds to wait=w527) -> ()  [unwired: 1 out]
                    }
                  }
                  n344 = property on="水平进度条" class="Slide (严格)"("Visible"=TRUE ("可见")) -> ()  [unwired: 2 in, 2 out]
                  n345 = flat-sequence {
                    tunnel: [w517] -> w497
                    frame #0 {
                      n346 = property on="X终点" class="DigNum (严格)"() -> ("Value"=w506:dbl)  [unwired: 2 in, 2 out]
                      n347 = property on="X起点" class="DigNum (严格)"() -> ("Value"=w505:dbl)  [unwired: 2 in, 2 out]
                      n348 = Subtract(x=w506, y=w505) -> (x-y=w510:dbl)
                      n349 = local read "X:"() -> (w509:dbl)
                      n350 = property on="X扫描范围" class="DigNum (严格)"("Value"=w510) -> ()  [unwired: 2 in, 2 out]
                      n351 = Divide(x=w510, y=w509) -> (x/y=w508:dbl)
                      n352 = Increment(x=w508) -> (x+1=w507:dbl)
                      n353 = property on="Xloop" class="DigNum (严格)"("Value"=w507) -> ()  [unwired: 2 in, 2 out]
                    }
                    frame #1 {
                      n354 = property on="Y终点" class="DigNum (严格)"() -> ("Value"=w512:dbl)  [unwired: 2 in, 2 out]
                      n355 = property on="Y起点" class="DigNum (严格)"() -> ("Value"=w511:dbl)  [unwired: 2 in, 2 out]
                      n356 = Subtract(x=w512, y=w511) -> (x-y=w515:dbl)
                      n357 = local read "Y:"() -> (w514:dbl)
                      n358 = property on="Y扫描范围" class="DigNum (严格)"("Value"=w515) -> ()  [unwired: 2 in, 2 out]
                      n359 = Divide(x=w515, y=w514) -> (x/y=w516:dbl)
                      n360 = Increment(x=w516) -> (x+1=w513:dbl)
                      n361 = property on="Yloop" class="DigNum (严格)"("Value"=w513) -> ()  [unwired: 2 in, 2 out]
                    }
                    frame #2 {
                      n362 = property on="Xloop" class="DigNum (严格)"() -> ("Value"=w520:dbl)  [unwired: 2 in, 2 out]
                      n363 = property on="Yloop" class="DigNum (严格)"() -> ("Value"=w517:dbl)  [unwired: 2 in, 2 out]
                      n364 = Initialize Array(0.0 ("元素"), w520, w517) -> (w519:dbl[][])
                      n365 = property on="强度图" class="IntGraph (严格)"("Value"=w519) -> ()  [unwired: 2 in, 2 out]
                    }
                  }
                  n366 = while {
                    shift-right: [w540] -> w500
                    shift-left: w498 -> [w540]
                    stop <- w545 stop-if-true
                    n367 = call "X,Y,Z轴坐标查询.vi"("细分设置"=8.0, "查询坐标轴"="Y", "串口通信端口"=w540) -> ("坐标(mm)"=w547:dbl)
                    n368 = property on="Y起点" class="DigNum (严格)"() -> ("Value"=w539:dbl)  [unwired: 2 in, 2 out]
                    n369 = property on="电机急停" class="Bool (严格)"() -> ("Value"=w546:bool)  [unwired: 2 in, 2 out]
                    n370 = Multiply(x=w547, y=1.0 ("x")) -> (x*y=w543:dbl)
                    n371 = Subtract(x=w539, y=w543) -> (x-y=w542:dbl)
                    n372 = case shown="真" w546 {
                      tunnel: w540 -> [_ w551]
                      frame False {
                      }
                      frame True {
                        n373 = call "步进电机命令输入与输出.vi"("输入字符串"="S0/", "串口通信端口"=w551) -> ()  [unwired: 1 out]
                      }
                    }
                    n374 = Absolute Value(x=w542) -> (abs(x)=w541:dbl)
                    n375 = local read "精度"() -> (w544:dbl)
                    n376 = property on="Y(mm)" class="DigNum (严格)"("Value"=w543) -> ()  [unwired: 2 in, 2 out]
                    n377 = Less?(x=w541, y=w544) -> (x < y?=w545:bool)
                  }
                  n378 = for {
                    N: w497 -> [_]
                    shift-right: [w589] -> _
                    shift-left: w501 -> [w589]
                    shift-right: [w588] -> _
                    shift-left: w503 -> [w588]
                    tunnel: [w587] -> w496 mode=indexing
                    shift-right: [w577] -> w495
                    shift-left: w500 -> [w579]
                    i -> [w572]
                    # "实时成像出问题调这里"
                    n379 = property on="Y序" class="DigNum (严格)"("Value"=w572) -> ()  [unwired: 2 in, 2 out]
                    n380 = local read "Yloop"() -> (w574:dbl)
                    n381 = Multiply(x=w574, y=0.01) -> (x*y=w573:dbl)
                    n382 = Divide(x=w572, y=w573) -> (x/y=w575:dbl)
                    n383 = property on="水平进度条" class="Slide (严格)"("Value"=w575) -> ()  [unwired: 2 in, 2 out]
                    n384 = flat-sequence {
                      tunnel: [w632] -> w592
                      tunnel: [w630] -> w591
                      tunnel: [w633] -> w587
                      tunnel: [w631] -> w590
                      tunnel: w579 -> [w629]
                      tunnel: [w663] -> w583
                      tunnel: w588 -> [w647]
                      tunnel: w589 -> [w646]
                      tunnel: w592 -> [w659]
                      tunnel: w591 -> [w663]
                      tunnel: w590 -> [w651]
                      frame #0 {
                        n385 = local read "精度"() -> (w641:dbl)
                        n386 = property on="细分设置" class="DigNum (严格)"() -> ("Value"=w640:dbl)  [unwired: 2 in, 2 out]
                        n387 = property on="X终点" class="DigNum (严格)"() -> ("Value"=w644:dbl)  [unwired: 2 in, 2 out]
                        n388 = property on="X起点" class="DigNum (严格)"() -> ("Value"=w628:dbl)  [unwired: 2 in, 2 out]
                        n389 = local read "pulDDR2Length"() -> (w636:u32)
                        n390 = local read "M_Length"() -> (w638:i32)
                        n391 = property on="hDevice" class="DigNum (严格)"() -> ("Value"=w637:i32)  [unwired: 2 in, 2 out]
                        n392 = property on="N_Length" class="DigNum (严格)"() -> ("Value"=w639:i32)  [unwired: 2 in, 2 out]
                        n393 = property on="等待时间" class="DigNum (严格)"() -> ("Value"=w642:u32)  [unwired: 2 in, 2 out]
                        n394 = property on="电机急停" class="Bool (严格)"() -> ("Value"=w643:bool)  [unwired: 2 in, 2 out]
                        n395 = call "X轴连续扫描（1.0）.vi"("VISA I"=w629, "X0"=w628, "X"=w644, "精度"=w641, "细分设置"=w640, "等待时间(ms)"=w642, "pulDDR2Length"=w636, "电机急停"=w643, "hDevice"=w637, "M-length"=w638, "N-length"=w639) -> ("VISA O"=w630:refnum<visa-resource-name>, "hDevice out"=w635:i32, "X"=w634:dbl, "强度图行"=w633:dbl[], "时域谱页"=w632:dbl[][], "幅频谱页"=w631:dbl[][])  [unwired: 3 in]
                        n396 = property on="hDevice 2" class="DigNum (严格)"("Value"=w635) -> ()  [unwired: 2 in, 2 out]
                        n397 = property on="X（mm）" class="DigNum (严格)"("Value"=w634) -> ()  [unwired: 2 in, 2 out]
                      }
                      frame #1 {
                        n398 = property on="Y序" class="DigNum (严格)"() -> ("Value"=w645:i32)  [unwired: 2 in, 2 out]
                        n399 = Increment(x=w645) -> (x+1=w648:i32)
                        n400 = Number To Decimal String(number=w648) -> (decimal integer string=w657:string)  [unwired: 1 in]
                        n401 = Number To Decimal String(number=w648) -> (decimal integer string=w656:string)  [unwired: 1 in]
                        n402 = Concatenate Strings("T" ("字符串"), w657, ".txt" ("字符串")) -> (w660:string)
                        n403 = Concatenate Strings("F" ("字符串"), w656, ".txt" ("字符串")) -> (w654:string)
                        n404 = Build Path(base path=w647, name or relative path=w660) -> (appended path=w662:path)
                        n405 = call-poly <vilib>:"Write Delimited Spreadsheet.vi"("file path (dialog if empty)"=w662, "2D data"=w659, "transpose? (no:F)"=FALSE) -> ()  [unwired: 11 in, 2 out]
                        n406 = Build Path(base path=w646, name or relative path=w654) -> (appended path=w652:path)
                        n407 = call-poly <vilib>:"Write Delimited Spreadsheet.vi"("file path (dialog if empty)"=w652, "2D data"=w651, "transpose? (no:F)"=FALSE) -> ()  [unwired: 11 in, 2 out]
                      }
                    }
                    n408 = flat-sequence {
                      tunnel: w583 -> [w605]
                      tunnel: [w605] -> w584
                      tunnel: [w604] -> w585
                      frame #0 {
                        n409 = property on="细分设置" class="DigNum (严格)"() -> ("Value"=w604:dbl)  [unwired: 2 in, 2 out]
                        n410 = Multiply(x=0.0, y=50.0) -> (x*y=w608:dbl)
                        n411 = Multiply(x=w608, y=w604) -> (x*y=w613:dbl)
                        n412 = local read "等待时间"() -> (w603:u32)
                        n413 = Number To Fractional String(number=w613, precision (6)=i16 0 ("精度(6)")) -> (F-format string=w611:string)  [unwired: 2 out]
                        n414 = Concatenate Strings("X=" ("字符串"), w611, "/" ("字符串")) -> (w606:string)
                        n415 = Wait (ms)(milliseconds to wait=w603) -> ()  [unwired: 1 out]
                        n416 = call "步进电机命令输入与输出.vi"("输入字符串"=w606, "串口通信端口"=w605) -> ()  [unwired: 1 out]
                      }
                    }
                    n417 = while {
                      shift-right: [w617] -> w582
                      shift-left: w584 -> [w617]
                      shift-right: [w615] -> _
                      shift-left: w585 -> [w615]
                      stop <- w621 stop-if-true
                      n418 = property on="电机急停" class="Bool (严格)"() -> ("Value"=w622:bool)  [unwired: 2 in, 2 out]
                      n419 = case shown="真" w622 {
                        tunnel: w617 -> [_ w626]
                        frame False {
                        }
                        frame True {
                          n420 = call "步进电机命令输入与输出.vi"("输入字符串"="S0/", "串口通信端口"=w626) -> ()  [unwired: 1 out]
                        }
                      }
                      n421 = call "X,Y,Z轴坐标查询.vi"("细分设置"=w615, "查询坐标轴"="X", "串口通信端口"=w617) -> ("坐标(mm)"=w623:dbl)
                      n422 = Multiply(x=w623, y=4.0 ("x")) -> (x*y=w619:dbl)
                      n423 = Subtract(x=0.0, y=w619) -> (x-y=w618:dbl)
                      n424 = local read "精度"() -> (w620:dbl)
                      n425 = Absolute Value(x=w618) -> (abs(x)=w616:dbl)
                      n426 = property on="X（mm）" class="DigNum (严格)"("Value"=w619) -> ()  [unwired: 2 in, 2 out]
                      n427 = Less?(x=w616, y=w620) -> (x < y?=w621:bool)
                    }
                    n428 = property on="强度图" class="IntGraph (严格)"() -> ("Value"=w595:dbl[][])  [unwired: 2 in, 2 out]
                    n429 = property on="Yloop" class="DigNum (严格)"() -> ("Value"=w580:dbl)  [unwired: 2 in, 2 out]
                    n430 = property on="Y序" class="DigNum (严格)"() -> ("Value"=w586:i32)  [unwired: 2 in, 2 out]
                    n431 = Replace Array Subset(array=w595, new element=w587, index (col)=w586) -> (w594:dbl[][])  [unwired: 1 in]
                    n432 = property on="强度图" class="IntGraph (严格)"("Value"=w594) -> ()  [unwired: 2 in, 2 out]
                    n433 = Decrement(x=w580) -> (x-1=w581:dbl)
                    n434 = Equal?(x=w586, y=w581) -> (x = y?=w593:bool)
                    n435 = case shown="真" w593 {
                      tunnel: w582 -> [w667 w697]
                      tunnel: [w665 w698] -> w578
                      frame False {
                        n436 = flat-sequence {
                          tunnel: w667 -> [w671]
                          tunnel: [w671] -> w666
                          tunnel: [w668] -> w664
                          frame #0 {
                            n437 = property on="细分设置" class="DigNum (严格)"() -> ("Value"=w668:dbl)  [unwired: 2 in, 2 out]
                            n438 = call "X,Y,Z轴坐标查询.vi"("细分设置"=w668, "查询坐标轴"="Y", "串口通信端口"=w671) -> ("坐标(mm)"=w672:dbl)
                            n439 = property on="Y:" class="DigNum (严格)"() -> ("Value"=w670:dbl)  [unwired: 2 in, 2 out]
                            n440 = Add(x=w672, y=w670) -> (x+y=w674:dbl)
                            "x+y 3" <- w674
                            n441 = Multiply(x=w674, y=200.0) -> (x*y=w678:dbl)
                            n442 = Multiply(x=w678, y=8.0 ("细分设置")) -> (x*y=w683:dbl)
                            n443 = Number To Fractional String(number=w683, precision (6)=i16 0 ("精度(6)")) -> (F-format string=w681:string)  [unwired: 2 out]
                            n444 = Concatenate Strings("Y=" ("字符串"), w681, "/" ("字符串")) -> (w676:string)
                            n445 = call "步进电机命令输入与输出.vi"("输入字符串"=w676, "串口通信端口"=w671) -> ()  [unwired: 1 out]
                            n446 = property on="等待时间" class="DigNum (严格)"() -> ("Value"=w669:u32)  [unwired: 2 in, 2 out]
                            n447 = Wait (ms)(milliseconds to wait=w669) -> ()  [unwired: 1 out]
                          }
                        }
                        n448 = while {
                          shift-right: [w686] -> w665
                          shift-left: w666 -> [w686]
                          shift-right: [w685] -> _
                          shift-left: w664 -> [w685]
                          stop <- w692 stop-if-true
                          n449 = call "X,Y,Z轴坐标查询.vi"("细分设置"=w685, "查询坐标轴"="Y", "串口通信端口"=w686) -> ("坐标(mm)"=w690:dbl)
                          n450 = property on="x+y 3" class="DigNum (严格)"() -> ("Value"=w684:dbl)  [unwired: 2 in, 2 out]
                          n451 = property on="电机急停" class="Bool (严格)"() -> ("Value"=w689:bool)  [unwired: 2 in, 2 out]
                          n452 = property on="Y(mm)" class="DigNum (严格)"("Value"=w690) -> ()  [unwired: 2 in, 2 out]
                          n453 = case shown="真" w689 {
                            tunnel: w686 -> [_ w694]
                            frame False {
                            }
                            frame True {
                              n454 = call "步进电机命令输入与输出.vi"("输入字符串"="S0/", "串口通信端口"=w694) -> ()  [unwired: 1 out]
                            }
                          }
                          n455 = Subtract(x=w684, y=w690) -> (x-y=w688:dbl)
                          n456 = Absolute Value(x=w688) -> (abs(x)=w687:dbl)
                          n457 = local read "精度"() -> (w691:dbl)
                          n458 = Less?(x=w687, y=w691) -> (x < y?=w692:bool)
                        }
                      }
                      frame True {
                        n459 = flat-sequence {
                          tunnel: [w702] -> _
                          tunnel: [w702] -> w699
                          tunnel: w697 -> [w702]
                          tunnel: [w700] -> w696
                          frame #0 {
                            n460 = property on="细分设置" class="DigNum (严格)"() -> ("Value"=w700:dbl)  [unwired: 2 in, 2 out]
                            n461 = Multiply(x=0.0, y=200.0) -> (x*y=w706:dbl)
                            n462 = Multiply(x=w706, y=w700) -> (x*y=w711:dbl)
                            n463 = Number To Fractional String(number=w711, precision (6)=i16 0 ("精度(6)")) -> (F-format string=w709:string)  [unwired: 2 out]
                            n464 = Concatenate Strings("Y=" ("字符串"), w709, "/" ("字符串")) -> (w704:string)
                            n465 = call "步进电机命令输入与输出.vi"("输入字符串"=w704, "串口通信端口"=w702) -> ()  [unwired: 1 out]
                            n466 = property on="等待时间" class="DigNum (严格)"() -> ("Value"=w701:u32)  [unwired: 2 in, 2 out]
                            n467 = Wait (ms)(milliseconds to wait=w701) -> ()  [unwired: 1 out]
                          }
                        }
                        n468 = while {
                          shift-right: [w713] -> w698
                          shift-left: w699 -> [w713]
                          shift-right: [w712] -> _
                          shift-left: w696 -> [w712]
                          stop <- w719 stop-if-true
                          n469 = property on="电机急停" class="Bool (严格)"() -> ("Value"=w720:bool)  [unwired: 2 in, 2 out]
                          n470 = call "X,Y,Z轴坐标查询.vi"("细分设置"=w712, "查询坐标轴"="Y", "串口通信端口"=w713) -> ("坐标(mm)"=w721:dbl)
                          n471 = case shown="真" w720 {
                            tunnel: w713 -> [_ w724]
                            frame False {
                            }
                            frame True {
                              n472 = call "步进电机命令输入与输出.vi"("输入字符串"="S0/", "串口通信端口"=w724) -> ()  [unwired: 1 out]
                            }
                          }
                          n473 = Multiply(x=w721, y=1.0 ("x")) -> (x*y=w717:dbl)
                          n474 = Subtract(x=w717, y=0.0 ("x")) -> (x-y=w715:dbl)
                          n475 = local read "精度"() -> (w718:dbl)
                          n476 = Absolute Value(x=w715) -> (abs(x)=w714:dbl)
                          n477 = property on="Y(mm)" class="DigNum (严格)"("Value"=w717) -> ()  [unwired: 2 in, 2 out]
                          n478 = Less?(x=w714, y=w718) -> (x < y?=w719:bool)
                        }
                      }
                    }
                    n479 = flat-sequence {
                      tunnel: w578 -> [w596]
                      tunnel: [w596] -> w577
                      frame #0 {
                        n480 = local read "毫秒计时值"() -> (w597:u32)
                        n481 = Tick Count (ms)() -> (millisecond timer value=w600:u32)
                        n482 = Subtract(x=w600, y=w597) -> (x-y=w598:u32)
                        n483 = Multiply(x=w598, y=0.001) -> (x*y=w601:dbl)
                        n484 = property on="已用时（s）" class="DigNum (严格)"("Value"=w601) -> ()  [unwired: 2 in, 2 out]
                      }
                    }
                  }
                  n485 = property on="已用时（s）" class="DigNum (严格)"("Visible"=TRUE ("可见")) -> ()  [unwired: 2 in, 2 out]
                  n486 = flat-sequence {
                    tunnel: w496 -> [w554]
                    tunnel: w495 -> [w555]
                    tunnel: [w555] -> w492
                    tunnel: [w554] -> w491
                    tunnel: [w557] -> w502
                    tunnel: w492 -> [w557]
                    tunnel: w491 -> [w558]
                    frame #0 {
                      n487 = property on="水平进度条" class="Slide (严格)"("Value"=u8 100 ("水平进度条")) -> ()  [unwired: 2 in, 2 out]
                    }
                    frame #1 {
                      n488 = local read "毫秒计时值"() -> (w562:u32)
                      n489 = property on="数组" class="Arr (严格)"("Value"=w558) -> ()  [unwired: 2 in, 2 out]
                      n490 = Transpose 2D Array(2D array=w558) -> (transposed array=w559:dbl[][])
                      n491 = Tick Count (ms)() -> (millisecond timer value=w563:u32)
                      n492 = property on="强度图" class="IntGraph (严格)"("Value"=w559) -> ()  [unwired: 2 in, 2 out]
                      n493 = Subtract(x=w563, y=w562) -> (x-y=w560:u32)
                      n494 = Multiply(x=w560, y=0.001) -> (x*y=w556:dbl)
                      n495 = property on="已用时（s）" class="DigNum (严格)"("Value"=w556) -> ()  [unwired: 2 in, 2 out]
                    }
                  }
                }
                event "分层图查看": Value Change {
                  n496 = event-data() -> ()  [unwired: 1 in, 6 out]
                  n497 = call "分层图显示1.1.vi"("IN"=w727) -> ("OUT"=w726:string)  [unwired: 10 in]
                }
              }
            }
          }
        }
        n498 = dll-call lib="PTH2]abs CUsersH301Desktopart闭环扫描程序采集卡控制INFamd64\nPCI8502_32" fn="PCI8502_ReleaseDeviceAD" label="ReleaseDeviceAD"("hDevice"="hDevice 2") -> ("hDevice"=w19:i32)  [unwired: 4 in, 2 out]
        n499 = VISA Close(VISA resource name=w17) -> (error out=→"错误输出":errorcluster)  [unwired: 1 in]
        n500 = dll-call lib="PTH2]abs CUsersH301Desktopart闭环扫描程序采集卡控制INFamd64\nPCI8502_32" fn="PCI8502_ReleaseDevice" label="ReleaseDevice"("hDevice"=w19) -> ()  [unwired: 5 in, 2 out]
        "M_Length" <- w23
      }
    }
  }
  n501 = property on="高级设置" class="Bool"("Visible"=FALSE ("可见")) -> ()  [unwired: 2 in, 2 out]
  n502 = property on="定位模式" class="Bool"("Visible"=FALSE ("可见")) -> ()  [unwired: 2 in, 2 out]
  n503 = property on="已用时（s）" class="DigNum (严格)"("Visible"=FALSE ("可见")) -> ()  [unwired: 2 in, 2 out]
